vi "RS232通信实验.vi"() -> ()   [LabVIEW 2011]
uses:
  <vilib>/STM32_DriverVI_Interface_F4/UART/UART Resource Name_F4.ctl
panel:
  out "串口字节数":u16
  in  "字符串 2":string
  out "字符串":string
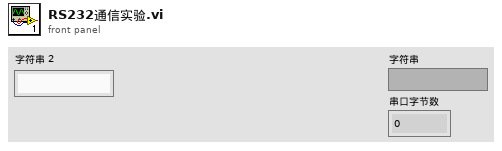
[diagram p1: front panel]
types:
  T1 = enum16{"1.0 bit", "0.5 bit", "2.0 bit", "1.5 bit"}
  T2 = enum16{"None parity", "Odd parity", "Even parity"}
  T3 = typedef "UART Resource Name_F4.ctl" = enum8{"COM 1", "COM 2", "COM 3", "COM 4", "COM 5", "COM 6"}
  T4 = typedef "STM32时钟倍频_F4.ctl" = u8
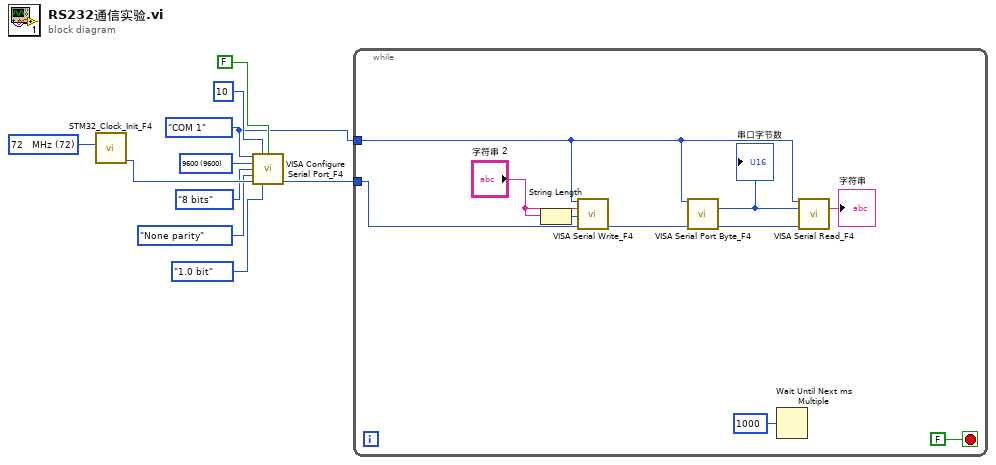
[diagram p0: block diagram]
diagram:
  w8 = u32 9600 items=["4800"=4800, "9600"=9600, "14400"=14400, "19200"=19200, "38400"=38400, "115200"=115200] ("baud rate (9600)")
  w1 = UART_Resource_Name_F4."COM 1" ("VISA resource name")
  w10 = T4 72 items=["32   MHz"=32, "72   MHz"=72, "120 MHz"=120, "168 MHz"=168, "216 MHz"=216] ("STM32F4时钟倍频")
  n1 = call <vilib>:"STM32_Clock_Init_F4.vi"("STM32F4时钟倍频"=w10) -> ("err_out"=w9:u8)  [unwired: 10 in]
  n2 = call <vilib>:"VISA Configure Serial Port_F4.vi"("VISA resource name"=w1, "termination char\n(0xA = '\\n' = LF)"=u8 10 ("termination char\n(0xA = '\\n' = LF)"), "Enable Termination Char (T)"=FALSE, "baud rate (9600)"=w8, "data bits (8)"=enum16{"8 bits", "9 bits"}."8 bits", "parity (0:none)"=T2."None parity", "err in"=w9, "stop bits (10: 1 bit)"=T1."1.0 bit") -> ("err out"=w2:u8)  [unwired: 7 in]
  n3 = while {
    tunnel: w2 -> [w18]
    tunnel: w1 -> [w15]
    stop <- FALSE stop-if-true
    n4 = String Length(string="字符串 2") -> (length=w12:i32)
    n5 = call <vilib>:"VISA Serial Write_F4.vi"("VISA resource name"=w15, "字符串"="字符串 2", "写入字节数"=w12, "err in"=w18) -> ("err out"=w17:u8)  [unwired: 11 in]
    n6 = call <vilib>:"VISA Serial Port Byte_F4.vi"("VISA resource name"=w15, "err in"=w17) -> ("串口字节数"=w14:u16, "err out"=w16:u8)  [unwired: 12 in]
    "串口字节数" <- w14
    n7 = Wait Until Next ms Multiple(millisecond multiple=u32 1000 ("毫秒倍数")) -> ()  [unwired: 1 out]
    n8 = call <vilib>:"VISA Serial Read_F4.vi"("VISA resource name"=w15, "读取字节数"=w14, "err in"=w16) -> ("字符串"=→"字符串":string)  [unwired: 10 in, 2 out]
  }
